vi "Check Connection.vi"(8 "error in (no error)":errorcluster, 11 "Instrument.lvclass in":refnum<class "Instrument.lvclass">) -> (0 "error out":errorcluster, 2 "connected?":bool, 3 "Instrument.lvclass out":refnum<class "Instrument.lvclass">)   [LabVIEW 2017, in "Instrument.lvclass"]
uses:
  Instrument.lvclass
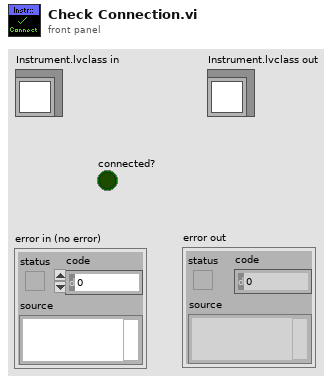
[diagram p1: front panel]
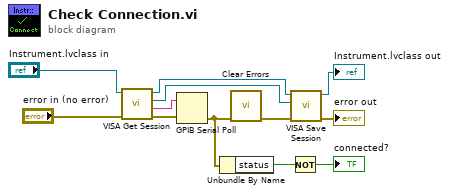
[diagram p0: block diagram]
diagram:
  n1 = call-dynamic "VISA Get Session.vi"("error in (no error)"="error in (no error)", "Instrument.lvclass in"="Instrument.lvclass in") -> ("error out"=w4:errorcluster, "GPIB string"=w5:string, "VISA Resource Name"=w1:refnum<visa-resource-name>, "Instrument.lvclass out"=w6:refnum<class "Instrument.lvclass">)  [unwired: 6 out]
  n2 = GPIB Serial Poll(0:w5, 1:w4) -> (4:w12:errorcluster)  [unwired: 2 out]
  n3 = Unbundle By Name(w12) -> ("status"=w11:bool)
  n4 = call <vilib>:"Clear Errors.vi"("error in (no error)"=w12) -> ("error out"=w7:errorcluster)  [unwired: 5 in, 1 out]
  n5 = Not(x=w11) -> (.not. x?=→"connected?":bool)
  n6 = call-dynamic "VISA Save Session.vi"("error in (no error)"=w7, "VISA Resource Name"=w1, "Instrument.lvclass in"=w6) -> ("error out"=→"error out":errorcluster, "Instrument.lvclass out"=→"Instrument.lvclass out":refnum<class "Instrument.lvclass">)  [unwired: 7 out]
